vi "실습 4-2.vi"() -> ()   [LabVIEW 2014]
panel:
  in  "가운데로":bool
  in  "메뉴바/도구바":bool
  in  "난수 발생":bool
  in  "경로":path
  out "웨이브폼 차트":dbl(graph)
  in  "정지":bool
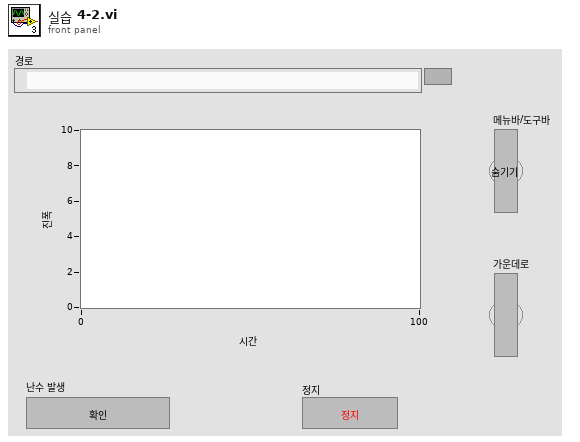
[diagram p1: front panel]
types:
  T1 = cluster{"left":i16, "top":i16, "right":i16, "bottom":i16}
  T2 = typedef "imagedata.ctl" = cluster{"image type":i32, "image depth":i32, "image":u8[], "mask":u8[], "colors":u32[], "Rectangle":cluster{"left":i16, "top":i16, "right":i16, "bottom":i16}}
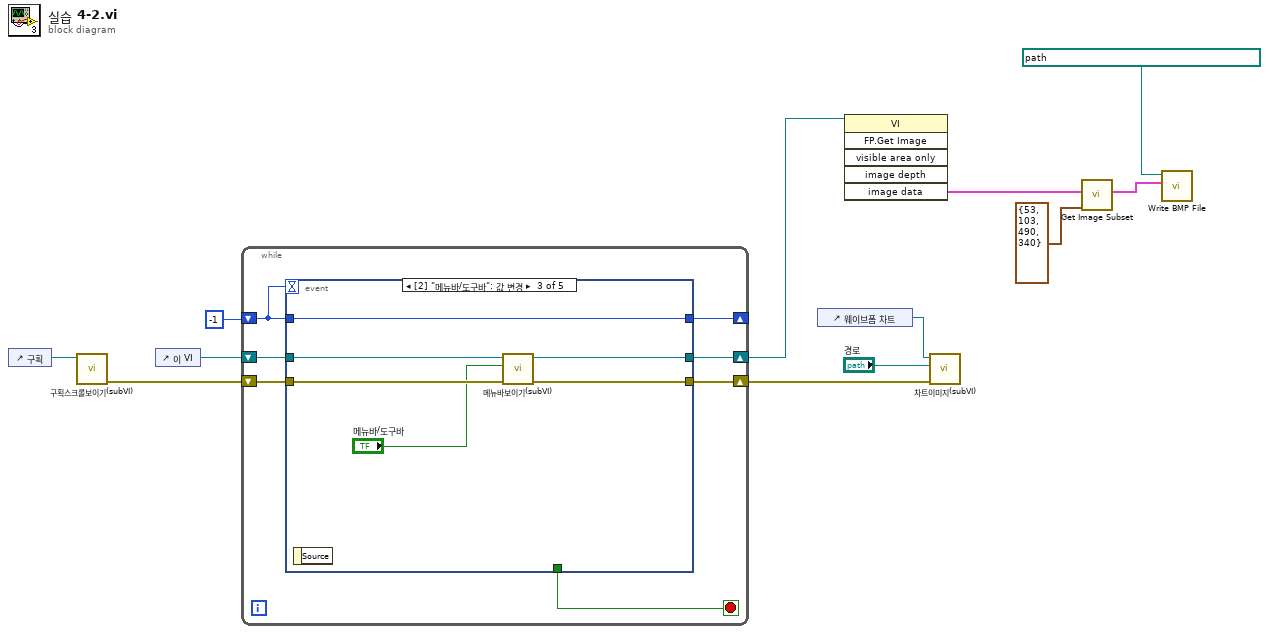
[diagram p0: block diagram]
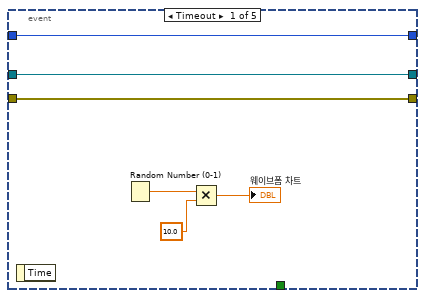
[diagram p2: hidden frame]
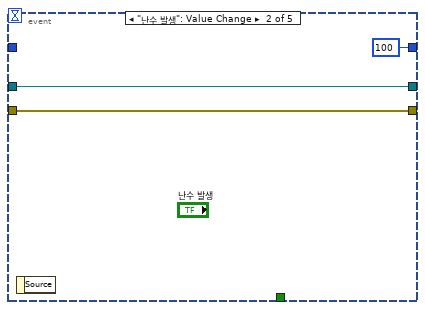
[diagram p3: hidden frame]
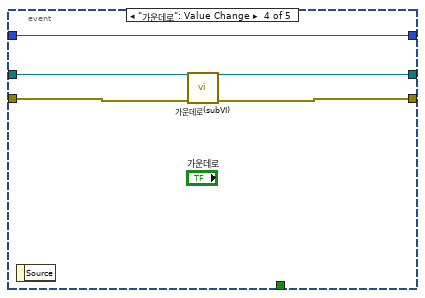
[diagram p4: hidden frame]
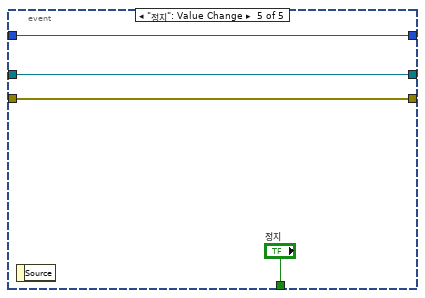
[diagram p5: hidden frame]
diagram:
  n1 = control-ref of="구획"() -> (w2:refnum<vi>)
  n2 = call "구획스크롤보이기(subVI).vi"("Pane 입력"=w2) -> ("에러 출력"=w10:errorcluster)  [unwired: 10 in]
  n3 = control-ref of="이 VI"() -> (w9:refnum<vi>)
  n4 = while {
    shift-right: [w18] -> _
    shift-left: -1 -> [w19]
    shift-right: [w16] -> w7
    shift-left: w10 -> [w17]
    shift-right: [w14] -> w6
    shift-left: w9 -> [w15]
    stop <- w13 stop-if-true
    n5 = event shown="[2] \"메뉴바/도구바\": 값 변경" {
      selector: _ -> [_ _ _ _ _]
      dyn-events: _ -> [_ _ _ _ _]
      timeout: w19 -> [_ _ _ _ _]
      tunnel: w19 -> [w25 _ w29 w35 w41]
      tunnel: [w25 100 w29 w35 w41] -> w18
      tunnel: w17 -> [w21 w28 w32 w37 w43]
      tunnel: [w21 w28 w30 w36 w43] -> w16
      tunnel: w15 -> [w20 w27 w34 w39 w42]
      tunnel: [w20 w27 w33 w38 w42] -> w14
      tunnel: [_ _ _ _ "정지"] -> w13
      event Timeout {
        n6 = event-data() -> ()  [unwired: 1 in, 1 out]
        n7 = Random Number (0-1)() -> (number: 0 to 1=w24:dbl)
        n8 = Multiply(x=w24, y=10.0) -> (x*y=→"웨이브폼 차트":dbl)
      }
      event "난수 발생": Value Change {
        n9 = event-data() -> ()  [unwired: 1 in, 1 out]
      }
      event "메뉴바/도구바": Value Change {
        n10 = event-data() -> ()  [unwired: 1 in, 1 out]
        n11 = call "메뉴바보이기(subVI).vi"("에러 입력(에러 없음)"=w32, "메뉴바/도구바"="메뉴바/도구바", "VI 입력"=w34) -> ("에러 출력"=w30:errorcluster, "VI 출력"=w33:refnum<vi>)  [unwired: 7 in]
      }
      event "가운데로": Value Change {
        n12 = event-data() -> ()  [unwired: 1 in, 1 out]
        n13 = call "가운데로(subVI).vi"("에러 입력(에러 없음)"=w37, "VI 입력"=w39) -> ("에러 출력"=w36:errorcluster, "VI 출력"=w38:refnum<vi>)  [unwired: 8 in]
      }
      event "정지": Value Change {
        n14 = event-data() -> ()  [unwired: 1 in, 1 out]
      }
    }
  }
  n15 = control-ref of="웨이브폼 차트"() -> (w1:refnum<vi>)
  n16 = invoke class="VI" method="FP.Get Image"(reference=w6) -> ("image data"=w5:T2)  [unwired: 5 in, 5 out]
  n17 = call "차트이미지(subVI).vi"("에러 입력(에러 없음)"=w7, "경로"="경로", "WaveformChart 입력"=w1) -> ()  [unwired: 9 in]
  n18 = call <vilib>:"Get Image Subset.vi"("subset rect"=T1 {"left"=53, "top"=103, "right"=490, "bottom"=340}, "image data"=w5) -> ("image subset"=w3:T2)  [unwired: 4 in, 1 out]
  n19 = call <vilib>:"Write BMP File.vi"("image data"=w3, "path to BMP file"=path "C:/Users/lvedu/Desktop/전체그림.BMP" ("경로 2")) -> ()  [unwired: 8 in, 2 out]
